vi "data-phase-ttl-extraction demo.vi"() -> ()   [LabVIEW 2009]
uses:
  <vilib>/Utility/file.llb/Read From Spreadsheet File (DBL).vi
panel:
  in  "TTL row index":i32=3
  in  "Phase row index":i32=1
  out "Phase Array":dbl[](array[numeric])
  out "all rows":dbl[][](array[numeric]) format="%0.3f"
  out "Waveform Graph":dbl[][](graph)
  in  "Path":path=path "F:/data/tomo/data-ttl.txt"
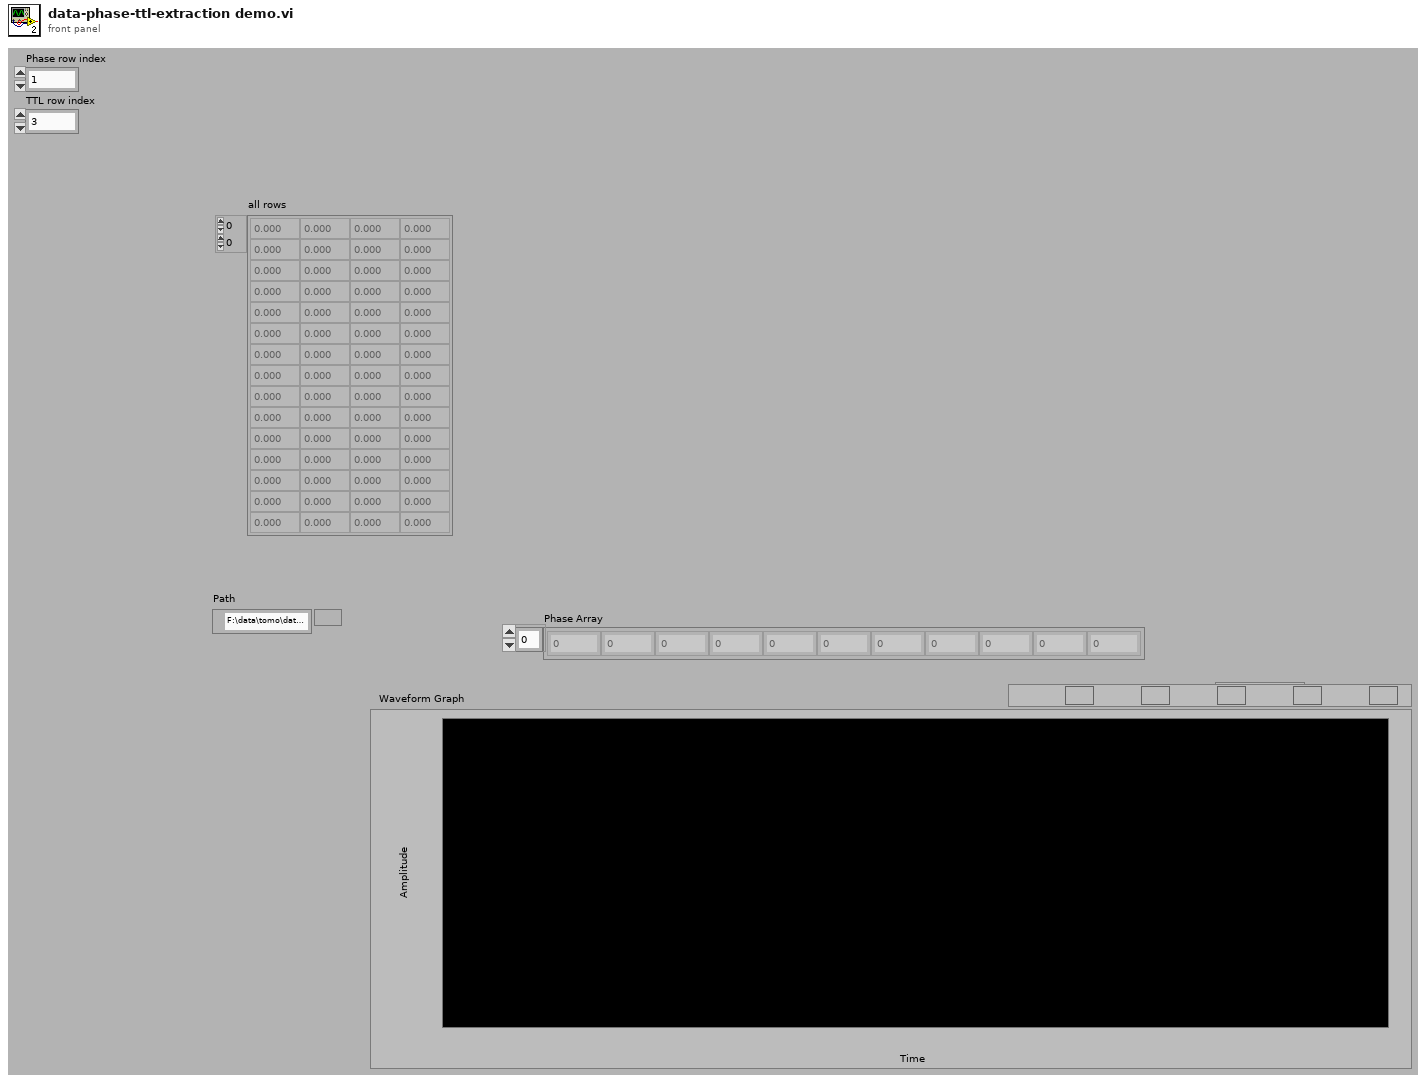
[diagram p1: front panel]
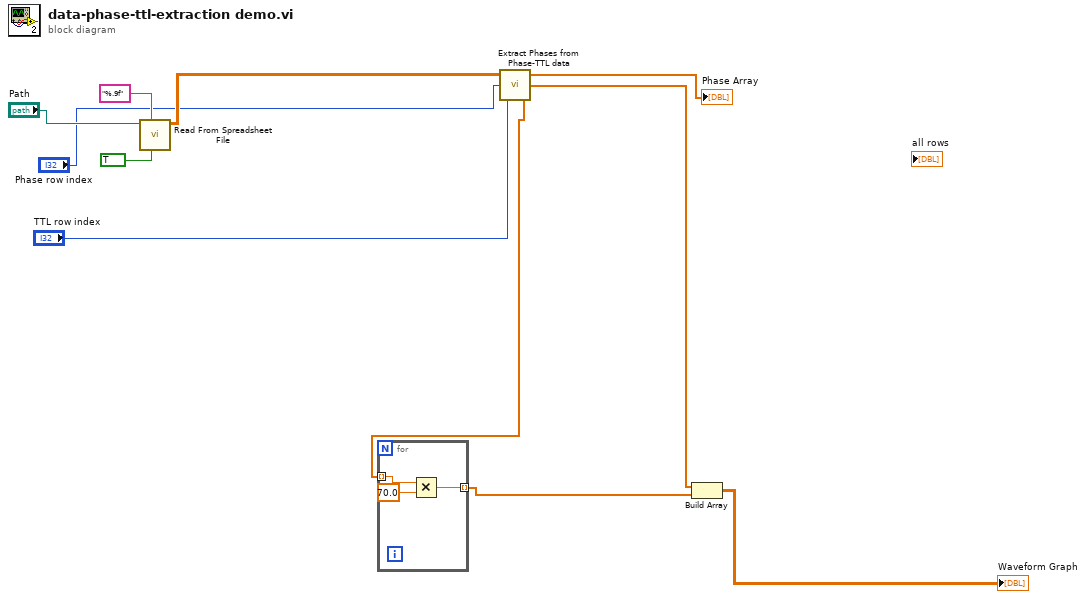
[diagram p0: block diagram]
diagram:
  n1 = call-poly <vilib>:"Read From Spreadsheet File.vi"("transpose (no:F)"=TRUE, "format (%.3f)"="%.9f", "file path (dialog if empty)"="Path") -> ("all rows"=w7:dbl[][])  [unwired: 4 in, 4 out]
  n2 = call "Extract Phases from Phase-TTL data.vi"("TTL row index"="TTL row index", "Phase row index"="Phase row index", "Phase-TTL Data"=w7) -> ("Input TTL array"=w3:dbl[], "Input Phase Array"=w2:dbl[], "Extracted Phases"=→"Phase Array":dbl[])
  n3 = for {
    tunnel: w3 -> [w14] mode=indexing
    tunnel: [w12] -> w4 mode=indexing
    n4 = Multiply(x=w14, y=70.0) -> (x*y=w12:dbl)
  }
  n5 = Build Array(w2, w4) -> (→"Waveform Graph":dbl[][])
